vi "Find All Minima 1D Inner Part (VI).vi"(4 "sign":i32(ring) items=["y=f(x)", "y=-f(x)"], 5 "accuracy":dbl=1e-08 format="%.2e", 6 "data":variant, 7 "f(x)":T1, 8 "end":dbl=1.0 format="%.2f", 9 "start":dbl format="%.2f", 10 "algorithm":u16(ring) items=["Golden Section Search", "Brent with Derivatives"], 11 "step type":u16(ring) items=["fixed function", "modified function"]) -> (0 "error out":i32, 1 "ticks":u32, 2 "f(Minima)":dbl[](array[numeric]) format="%.2f", 3 "Minima":dbl[](array[numeric]) format="%.2f")   [LabVIEW 2017, in "NI_Gmath.lvlib"]
uses:
  <vilib>/gmath/NI_Gmath.lvlib
  <vilib>/gmath/_ref_NR.llb/functionRefnum.ctl
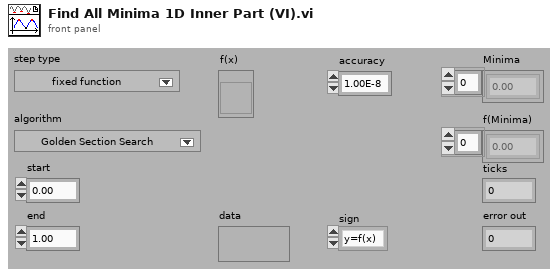
[diagram p1: front panel]
types:
  T1 = typedef "NI_Gmath.lvlib/functionRefnum.ctl" = refnum<vi>
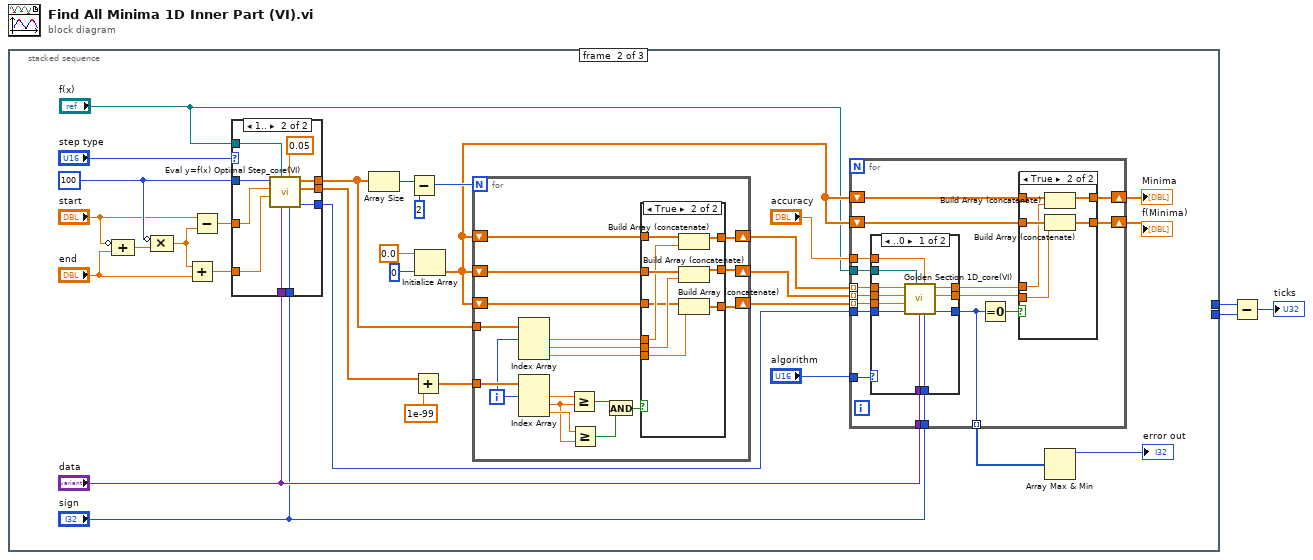
[diagram p0: block diagram]
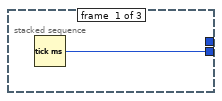
[diagram p2: hidden frame]
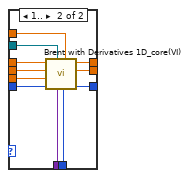
[diagram p4: hidden frame]
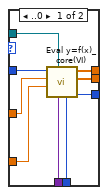
[diagram p6: hidden frame]
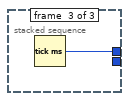
[diagram p7: hidden frame]
diagram:
  n1 = stacked-sequence {
    tunnel: [w4 _ _] -> w2
    tunnel: [_ _ w132] -> w3
    frame #0 {
      n2 = Tick Count (ms)() -> (millisecond timer value=w4:u32)
    }
    frame #1 {
      w31 = u32 100
      n3 = Compound Arithmetic op=ADD(invert "start", "end") -> (w30:dbl)
      n4 = Compound Arithmetic op=MULTIPLY(invert w31, w30) -> (w26:dbl)
      n5 = Add(x=w26, y="end") -> (x+y=w28:dbl)
      n6 = Subtract(x="start", y=w26) -> (x-y=w25:dbl)
      n7 = case shown="1.." "step type" {
        tunnel: w31 -> [w119 w131]
        tunnel: w25 -> [w118 w125]
        tunnel: w28 -> [w117 w124]
        tunnel: [w120 w129] -> w11
        tunnel: [w121 w130] -> w12
        tunnel: "f(x)" -> [w114 w123]
        tunnel: "data" -> [w115 w128]
        tunnel: [w116 w127] -> w8
        tunnel: "sign" -> [w113 w122]
        frame ..0 {
          n8 = call <vilib>:"Eval y=f(x)_core(VI).vi"("sign"=w113, "data"=w115, "f(x)"=w114, "end"=w117, "start"=w118, "number of points"=w119) -> ("error out"=w116:i32, "Y Values"=w120:dbl[], "X Values"=w121:dbl[])  [unwired: 2 in, 1 out]
        }
        frame 1.. {
          n9 = call <vilib>:"Eval y=f(x) Optimal Step_core(VI).vi"("sign"=w122, "epsilon"=0.05, "data"=w128, "f(x)"=w123, "end"=w124, "start"=w125, "number of points"=w131) -> ("error out"=w127:i32, "Y Values"=w129:dbl[], "X Values"=w130:dbl[])  [unwired: 1 in, 1 out]
        }
      }
      n10 = Array Size(array=w12) -> (size(s)=w19:i32)
      n11 = Subtract(x=w19, y=2) -> (x-y=w18:i32)
      n12 = Add(x=w11, y=1e-99) -> (x+y=w16:dbl[])
      n13 = Initialize Array(0.0, 0) -> (w9:dbl[])
      n14 = for {
        N: w18 -> [_]
        tunnel: w16 -> [w87]
        shift-right: [w99] -> w21
        shift-left: w9 -> [w100]
        shift-right: [w97] -> w20
        shift-left: w9 -> [w98]
        tunnel: w12 -> [w91]
        shift-right: [w95] -> w15
        shift-left: w9 -> [w96]
        i -> [w83]
        n15 = Index Array(array=w91, index #1=w83) -> (element #1=w90:dbl, element #2=w89:dbl, element #3=w88:dbl)  [unwired: 2 in]
        n16 = Index Array(array=w87, index #1=w83) -> (element #1=w86:dbl, element #2=w84:dbl, element #3=w85:dbl)  [unwired: 2 in]
        n17 = Greater Or Equal?(x=w86, y=w84) -> (x >= y?=w94:bool)
        n18 = Greater Or Equal?(x=w85, y=w84) -> (x >= y?=w93:bool)
        n19 = And(x=w94, y=w93) -> (x .and. y?=w92:bool)
        n20 = case shown="True" w92 {
          tunnel: w100 -> [w103 w112]
          tunnel: [w103 w111] -> w99
          tunnel: w98 -> [w102 w110]
          tunnel: [w102 w109] -> w97
          tunnel: w90 -> [_ w108]
          tunnel: w89 -> [_ w107]
          tunnel: w96 -> [w101 w106]
          tunnel: [w101 w105] -> w95
          tunnel: w88 -> [_ w104]
          frame False {
          }
          frame True {
            n21 = Build Array (concatenate)(w112, w108) -> (w111:dbl[])
            n22 = Build Array (concatenate)(w110, w107) -> (w109:dbl[])
            n23 = Build Array (concatenate)(w106, w104) -> (w105:dbl[])
          }
        }
      }
      n24 = for {
        tunnel: w21 -> [w39] mode=indexing
        tunnel: w20 -> [w37] mode=indexing
        shift-right: [w48] -> w33
        shift-left: w9 -> [w52]
        shift-right: [w44] -> w32
        shift-left: w9 -> [w50]
        tunnel: w15 -> [w47] mode=indexing
        tunnel: "accuracy" -> [w46]
        tunnel: "algorithm" -> [w45]
        tunnel: [w40] -> w13 mode=indexing
        tunnel: "f(x)" -> [w42]
        tunnel: "data" -> [w41]
        tunnel: w8 -> [w38]
        tunnel: "sign" -> [w36]
        n25 = case shown="..0" w45 {
          tunnel: w46 -> [w66 w76]
          tunnel: w47 -> [w64 w75]
          tunnel: [w70 w81] -> w49
          tunnel: [w71 w82] -> w51
          tunnel: [w69 w80] -> w40
          tunnel: w42 -> [w68 w79]
          tunnel: w41 -> [w67 w78]
          tunnel: w38 -> [w63 w74]
          tunnel: w39 -> [w65 w77]
          tunnel: w37 -> [w62 w73]
          tunnel: w36 -> [w61 w72]
          frame ..0 {
            n26 = call <vilib>:"Golden Section 1D_core(VI).vi"("sign"=w61, "accuracy"=w66, "data"=w67, "f(x)"=w68, "error in"=w63, "c (start)"=w64, "b (start)"=w62, "a (start)"=w65) -> ("error out"=w69:i32, "f(minimum)"=w70:dbl, "minimum"=w71:dbl)  [unwired: 1 out]
          }
          frame 1.. {
            n27 = call <vilib>:"Brent with Derivatives 1D_core(VI).vi"("sign"=w72, "accuracy"=w76, "data"=w78, "f(x)"=w79, "error in"=w74, "c (start)"=w75, "b (start)"=w73, "a (start)"=w77) -> ("error out"=w80:i32, "f(minimum)"=w81:dbl, "minimum"=w82:dbl)  [unwired: 1 out]
          }
        }
        n28 = Equal To 0?(x=w40) -> (x = 0?=w43:bool)
        n29 = case shown="True" w43 {
          tunnel: [w53 w60] -> w44
          tunnel: [w54 w59] -> w48
          tunnel: w49 -> [_ w58]
          tunnel: w50 -> [w53 w57]
          tunnel: w51 -> [_ w56]
          tunnel: w52 -> [w54 w55]
          frame False {
          }
          frame True {
            n30 = Build Array (concatenate)(w55, w56) -> (w59:dbl[])
            n31 = Build Array (concatenate)(w57, w58) -> (w60:dbl[])
          }
        }
      }
      "f(Minima)" <- w32
      "Minima" <- w33
      n32 = Array Max & Min(array=w13) -> (max value=→"error out":i32)  [unwired: 3 out]
    }
    frame #2 {
      n33 = Tick Count (ms)() -> (millisecond timer value=w132:u32)
    }
  }
  n34 = Subtract(x=w3, y=w2) -> (x-y=→"ticks":u32)
